vi "LJM_eReadNameArray.vi"(0 "Handle In":i32, 5 "Name":string, 11 "error in":errorcluster, 13 "NumValues":i32) -> (4 "Handle Out":i32, 10 "aValues":dbl[](array[numeric]) format="%.2f", 14 "ErrorAddress":i32, 15 "error out":errorcluster)   [LabVIEW 2020]
uses:
  LabJackM.framework
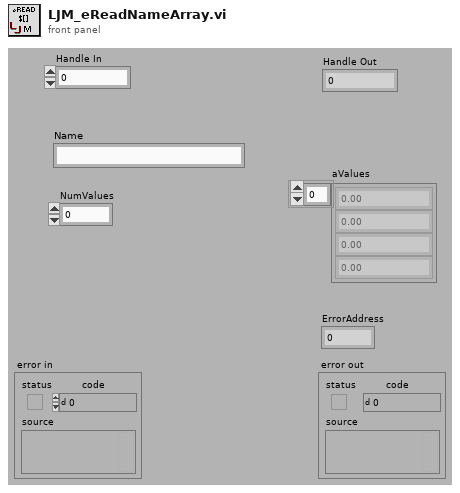
[diagram p1: front panel]
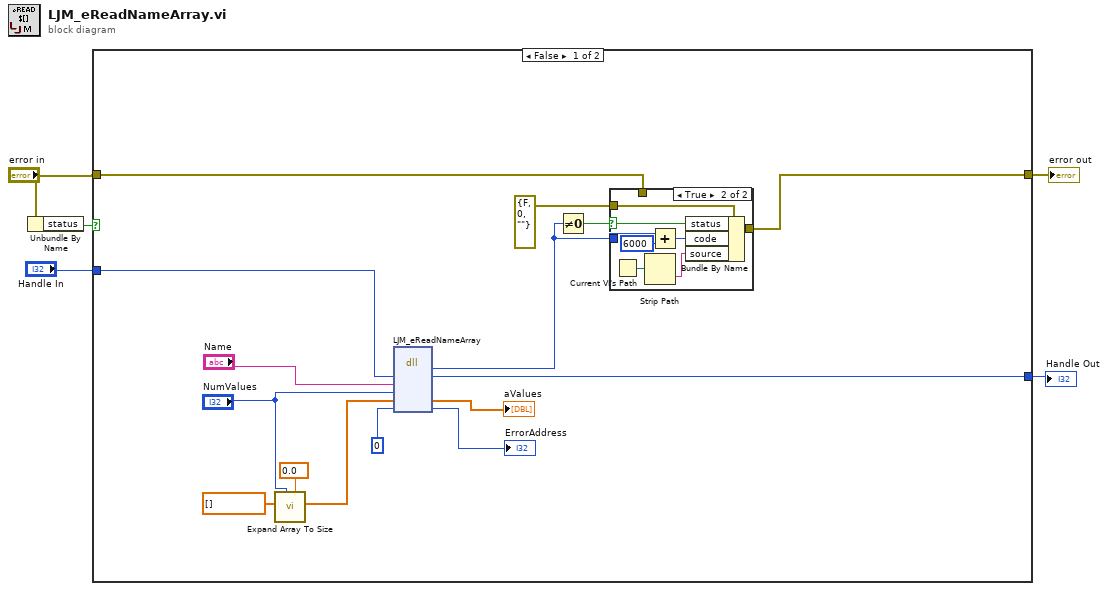
[diagram p0: block diagram]
diagram:
  n1 = Unbundle By Name("error in") -> ("status"=w5:bool)
  n2 = case shown="False" w5 {
    tunnel: "error in" -> [w17 w31]
    tunnel: [w16 w31] -> w2
    tunnel: [w13 w30] -> w1
    tunnel: "Handle In" -> [w12 w30]
    frame False {
      n3 = call "Expand Array To Size.vi"("Default Value"=0.0, "# Elements"="NumValues", "DBL Array In"=dbl[] []) -> ("DBL Array Out"=w10:dbl[])  [unwired: 4 in, 4 out]
      n4 = dll-call lib="LabJackM.framework" fn="LJM_eReadNameArray"("Handle"=w12, "Name"="Name", "NumValues"="NumValues", "aValues"=w10, "ErrorAddress"=u32 0 ("ErrorFrame")) -> ("return type"=w20:i32, "Handle"=w13:i32, "aValues"=→"aValues":dbl[], "ErrorAddress"=→"ErrorAddress":i32)  [unwired: 5 in, 2 out]
      n5 = Not Equal To 0?(x=w20) -> (x != 0?=w19:bool)
      n6 = case shown="True" w19 {
        selector: w19 -> [_ w28]
        tunnel: [w21 w29] -> w16
        tunnel: errorcluster {"status"=FALSE, "code"=0, "source"=""} ("error IO") -> [_ w27]
        tunnel: w20 -> [_ w23]
        tunnel: w17 -> [w21 _]
        frame False {
        }
        frame True {
          n7 = Current VI's Path() -> (path=w25:path)
          n8 = Strip Path(path=w25) -> (name=w26:string)  [unwired: 1 out]
          n9 = Add(x=w23, y=6000) -> (x+y=w24:i32)
          n10 = Bundle By Name(cluster=w27, "status"=w28, "code"=w24, "source"=w26) -> (w29:errorcluster)
        }
      }
    }
    frame True {
    }
  }
  "error out" <- w2
  "Handle Out" <- w1
